vi "PID Initializer.vi"(4 "CANCoder Can IDs":T1, 6 "Cancoder????":bool, 8 "error in":errorcluster, 10 "PIDF":cluster{"P":dbl, "I":dbl, "D":dbl, "F":dbl} {"F" format="%#_13g"; "D" format="%#_13g"; "I" format="%#_13g"; "P" format="%#_13g"}, 11 "Can IDs":T1) -> (0 "error out":errorcluster, 3 "Motors":T7)   [LabVIEW 2020]
uses:
  <vilib>/Rock Robotics/WPI/MotorControl/WPI_MotorControlDeviceRef.ctl
  <vilib>/Rock Robotics/WPI/MotorControl/WPI_MotorControlType.ctl
  <vilib>/Rock Robotics/SystemInterfaces/DIO/FPGA_DIOPWMChannel.ctl
  <vilib>/Rock Robotics/WPI/PWM/WPI_PWMDeadband.ctl
  <vilib>/Rock Robotics/SystemInterfaces/DIO/FPGA_DIOChannel.ctl
  <vilib>/Rock Robotics/WPI/ThirdParty/Phoenix-LabVIEW/Motor Controller/Controls/CTRE_Phoenix_MotorControl_NeutralMode.ctl
  <vilib>/Rock Robotics/WPI/ThirdParty/Phoenix-LabVIEW/Motor Controller/Controls/CTRE_Phoenix_MotorControl_FeedbackDevice_TalonFX.ctl
  <vilib>/Rock Robotics/WPI/ThirdParty/Phoenix-LabVIEW/Motor Controller/Controls/CTRE_Phoenix_MotorControl_RemoteSourceType.ctl
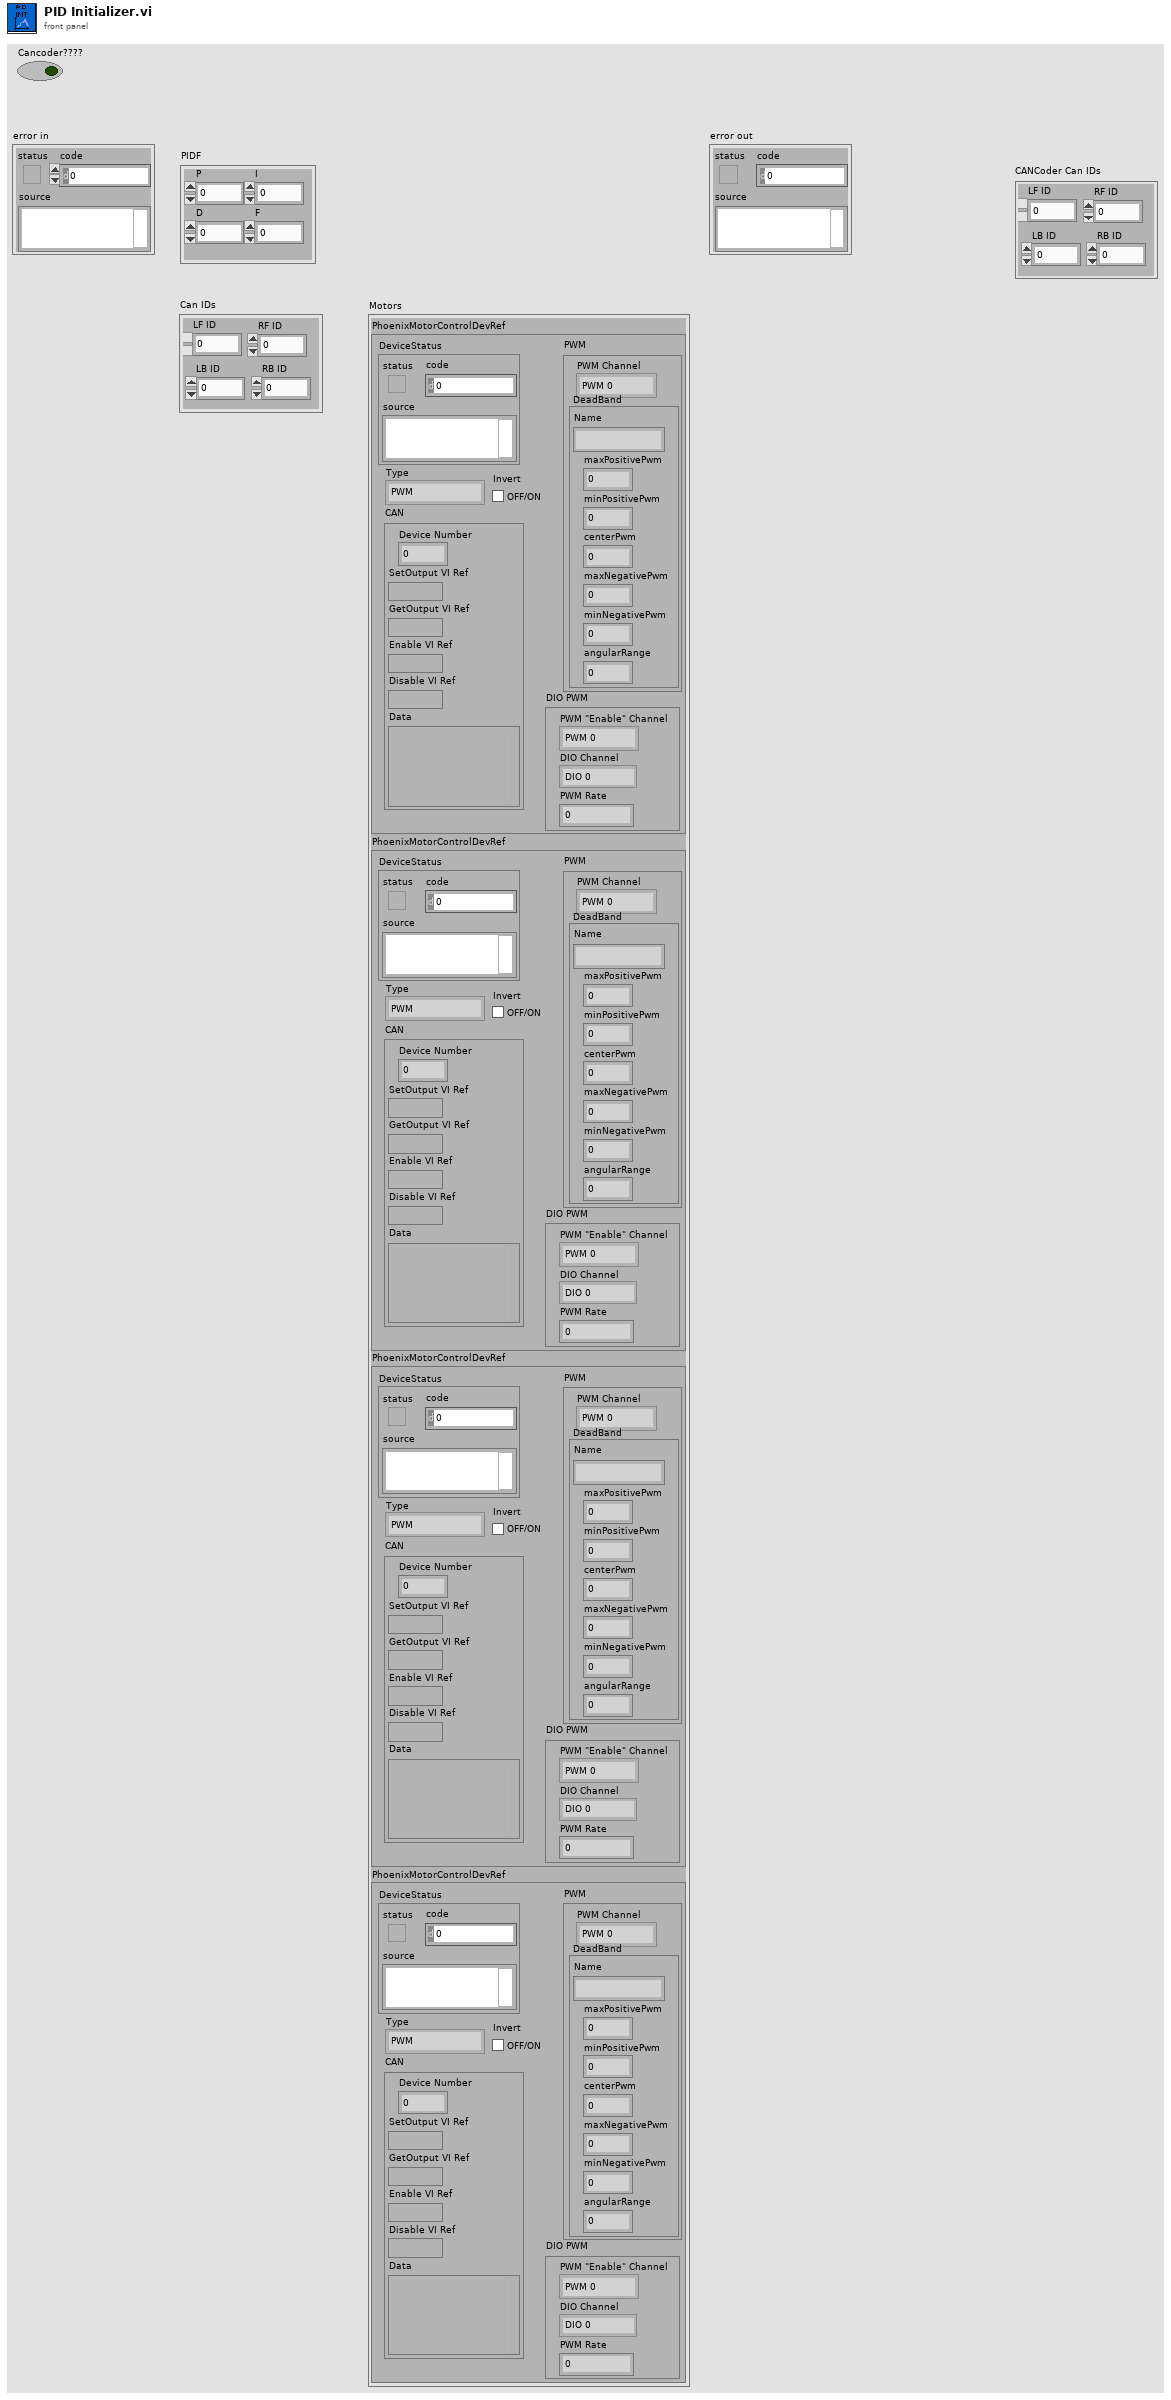
[diagram p1: front panel]
types:
  T1 = cluster{"LF ID":u8, "LB ID":u8, "RF ID":u8, "RB ID":u8}
  T2 = typedef "WPI_MotorControlDeviceRef.ctl" = cluster{"DeviceStatus":errorcluster, "Type":T3, "PWM":cluster{"PWM Channel":T4, "DeadBand":T5}, "CAN":cluster{"Device Number":u8, "SetOutput VI Ref":variant, "GetOutput VI Ref":variant, "Enable VI Ref":variant, "Disable VI Ref":variant, "Data":variant}, "Invert":bool, "DIO PWM":cluster{"PWM \"Enable\" Channel":T4, "DIOChannel":T6, "PWM Rate":dbl}}
  T3 = typedef "WPI_MotorControlType.ctl" = enum16{"PWM", "CAN", "DIO PWM"}
  T4 = typedef "FPGA_DIOPWMChannel.ctl" = enum8{"PWM 0", "PWM 1", "PWM 2", "PWM 3", "PWM 4", "PWM 5", "PWM 6", "PWM 7", "PWM 8", "PWM 9", "PWM MXP 0", "PWM MXP 1", "PWM MXP 2", "PWM MXP 3", "PWM MXP 4", "PWM MXP 5", "PWM MXP 6", "PWM MXP 7", "PWM MXP 8", "PWM MXP 9", "Invalid"}
  T5 = typedef "WPI_PWMDeadband.ctl" = cluster{"Name":string, "maxPositivePwm":i32, "minPositivePwm":i32, "centerPwm":i32, "maxNegativePwm":i32, "minNegativePwm":i32, "angularRange":u16}
  T6 = typedef "FPGA_DIOChannel.ctl" = enum8{"DIO 0", "DIO 1", "DIO 2", "DIO 3", "DIO 4", "DIO 5", "DIO 6", "DIO 7", "DIO 8", "DIO 9", "DIO MXP 0", "DIO MXP 1", "DIO MXP 2", "DIO MXP 3", "DIO MXP 4", "DIO MXP 5", "DIO MXP 6", "DIO MXP 7", "DIO MXP 8", "DIO MXP 9", "DIO MXP 10", "DIO MXP 11", "DIO MXP 12", "DIO MXP 13", "DIO MXP 14", "DIO MXP 15", "SPI Port CS1", "SPI Port CS2", "SPI Port CS3", "SPI Port MISO", "SPI Port MOSI", "Invalid"}
  T7 = cluster{"PhoenixMotorControlDevRef":T2, "PhoenixMotorControlDevRef":T2, "PhoenixMotorControlDevRef":T2, "PhoenixMotorControlDevRef":T2}
  T8 = typedef "CTRE_Phoenix_MotorControl_NeutralMode.ctl" = enum8{"EEPROMSetting", "Override to Coast", "Override to Brake"}
  T9 = typedef "CTRE_Phoenix_MotorControl_RemoteSourceType.ctl" = enum16{"Off", "Talon SRX Selected Sensor", "Pigeon IMU Yaw", "Pigeon IMU Pitch", "Pigeon IMU Roll", "CANifier Quadrature", "CANifier PWM Input 0", "CANifier PWM Input 1", "CANifier PWM Input 2", "CANifier PWM Input 3", "Gadgeteer Pigeon Yaw", "Gadgeteer Pigeon Pitch", "Gadgeteer Pigeon Roll", "CANCoder"}
  T10 = typedef "CTRE_Phoenix_MotorControl_FeedbackDevice_TalonFX.ctl" = i8
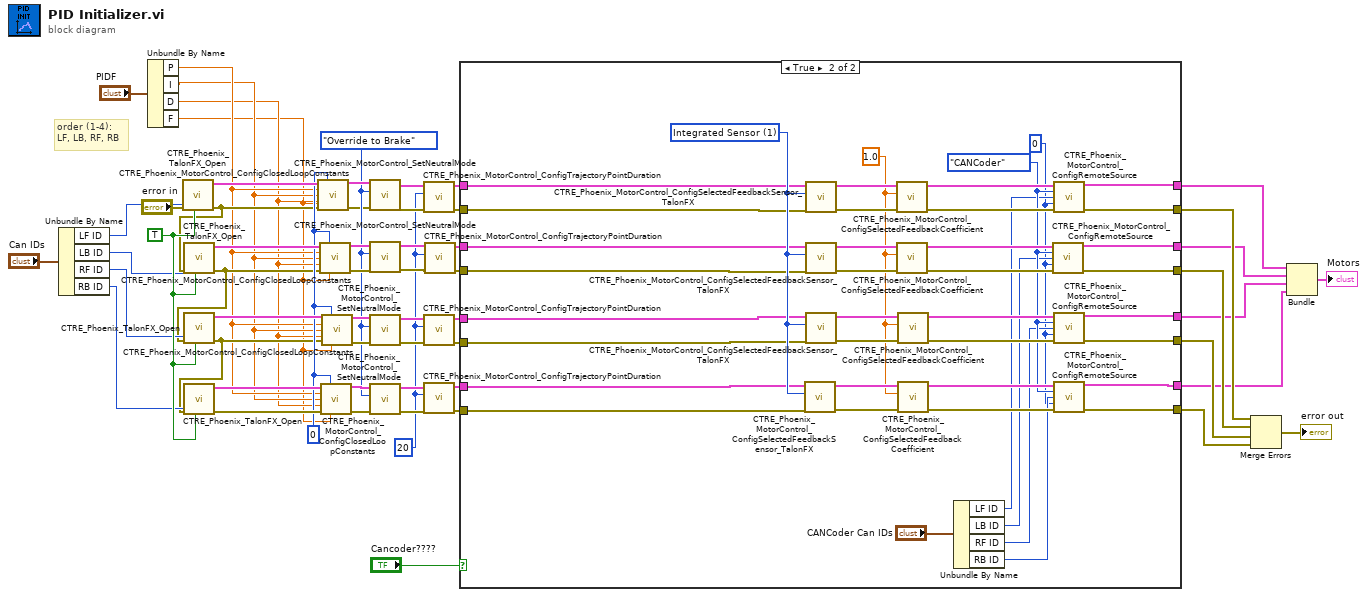
[diagram p0: block diagram]
diagram:
  w19 = 20 ("durationMs")
  w32 = CTRE_Phoenix_MotorControl_NeutralMode."Override to Brake" ("Motor Control Neutral Mode")
  w52 = 0 ("slotIdx")
  w53 = TRUE ("Invert")
  # "order (1-4):\nLF, LB, RF, RB"
  n1 = Unbundle By Name("Can IDs") -> ("LF ID"=w51:u8, "LB ID"=w50:u8, "RF ID"=w49:u8, "RB ID"=w48:u8)
  n2 = Unbundle By Name("PIDF") -> ("P"=w43:dbl, "I"=w42:dbl, "D"=w41:dbl, "F"=w40:dbl)
  n3 = call <vilib>:"CTRE_Phoenix_TalonFX_Open.vi"("Invert"=w53, "error in"="error in", "Device Number"=w51) -> ("error out"=w47:errorcluster, "PhoenixMotorControlDevRef"=w58:T2)  [unwired: 7 in]
  n4 = call <vilib>:"CTRE_Phoenix_TalonFX_Open.vi"("Invert"=w53, "error in"=w47, "Device Number"=w50) -> ("error out"=w46:errorcluster, "PhoenixMotorControlDevRef"=w57:T2)  [unwired: 7 in]
  n5 = call <vilib>:"CTRE_Phoenix_TalonFX_Open.vi"("Invert"=w53, "error in"=w46, "Device Number"=w49) -> ("error out"=w45:errorcluster, "PhoenixMotorControlDevRef"=w56:T2)  [unwired: 7 in]
  n6 = call <vilib>:"CTRE_Phoenix_TalonFX_Open.vi"("Invert"=w53, "error in"=w45, "Device Number"=w48) -> ("error out"=w54:errorcluster, "PhoenixMotorControlDevRef"=w55:T2)  [unwired: 7 in]
  n7 = call <vilib>:"CTRE_Phoenix_MotorControl_ConfigClosedLoopConstants.vi"("PhoenixMotorControlDevRef"=w58, "slotIdx"=w52, "P"=w43, "I"=w42, "D"=w41, "error in (no error)"=w47, "F"=w40) -> ("PhoenixMotorControlDevRef"=w33:T2, "error out"=w31:errorcluster)  [unwired: 7 in]
  n8 = call <vilib>:"CTRE_Phoenix_MotorControl_ConfigClosedLoopConstants.vi"("PhoenixMotorControlDevRef"=w57, "slotIdx"=w52, "P"=w43, "I"=w42, "D"=w41, "error in (no error)"=w46, "F"=w40) -> ("PhoenixMotorControlDevRef"=w37:T2, "error out"=w38:errorcluster)  [unwired: 7 in]
  n9 = call <vilib>:"CTRE_Phoenix_MotorControl_ConfigClosedLoopConstants.vi"("PhoenixMotorControlDevRef"=w55, "slotIdx"=w52, "P"=w43, "I"=w42, "D"=w41, "error in (no error)"=w54, "F"=w40) -> ("PhoenixMotorControlDevRef"=w34:T2, "error out"=w30:errorcluster)  [unwired: 7 in]
  n10 = call <vilib>:"CTRE_Phoenix_MotorControl_ConfigClosedLoopConstants.vi"("PhoenixMotorControlDevRef"=w56, "slotIdx"=w52, "P"=w43, "I"=w42, "D"=w41, "error in (no error)"=w45, "F"=w40) -> ("PhoenixMotorControlDevRef"=w35:T2, "error out"=w36:errorcluster)  [unwired: 7 in]
  n11 = call <vilib>:"CTRE_Phoenix_MotorControl_SetNeutralMode.vi"("error in (no error)"=w31, "Motor Control Neutral Mode"=w32, "PhoenixMotorControlDevRef"=w33) -> ("error out"=w21:errorcluster, "PhoenixMotorControlDevRef"=w20:T2)  [unwired: 7 in]
  n12 = call <vilib>:"CTRE_Phoenix_MotorControl_SetNeutralMode.vi"("error in (no error)"=w38, "Motor Control Neutral Mode"=w32, "PhoenixMotorControlDevRef"=w37) -> ("error out"=w22:errorcluster, "PhoenixMotorControlDevRef"=w23:T2)  [unwired: 7 in]
  n13 = call <vilib>:"CTRE_Phoenix_MotorControl_SetNeutralMode.vi"("error in (no error)"=w36, "Motor Control Neutral Mode"=w32, "PhoenixMotorControlDevRef"=w35) -> ("error out"=w24:errorcluster, "PhoenixMotorControlDevRef"=w25:T2)  [unwired: 7 in]
  n14 = call <vilib>:"CTRE_Phoenix_MotorControl_SetNeutralMode.vi"("error in (no error)"=w30, "Motor Control Neutral Mode"=w32, "PhoenixMotorControlDevRef"=w34) -> ("error out"=w26:errorcluster, "PhoenixMotorControlDevRef"=w27:T2)  [unwired: 7 in]
  n15 = call <vilib>:"CTRE_Phoenix_MotorControl_ConfigTrajectoryPointDuration.vi"("error in"=w21, "durationMs"=w19, "PhoenixMotorControlDevRef"=w20) -> ("error out"=w16:errorcluster, "PhoenixMotorControlDevRef"=w17:T2)  [unwired: 7 in]
  n16 = call <vilib>:"CTRE_Phoenix_MotorControl_ConfigTrajectoryPointDuration.vi"("error in"=w24, "durationMs"=w19, "PhoenixMotorControlDevRef"=w25) -> ("error out"=w12:errorcluster, "PhoenixMotorControlDevRef"=w13:T2)  [unwired: 7 in]
  n17 = call <vilib>:"CTRE_Phoenix_MotorControl_ConfigTrajectoryPointDuration.vi"("error in"=w26, "durationMs"=w19, "PhoenixMotorControlDevRef"=w27) -> ("error out"=w10:errorcluster, "PhoenixMotorControlDevRef"=w11:T2)  [unwired: 7 in]
  n18 = call <vilib>:"CTRE_Phoenix_MotorControl_ConfigTrajectoryPointDuration.vi"("error in"=w22, "durationMs"=w19, "PhoenixMotorControlDevRef"=w23) -> ("error out"=w14:errorcluster, "PhoenixMotorControlDevRef"=w15:T2)  [unwired: 7 in]
  n19 = case shown="True" "Cancoder????" {
    tunnel: w17 -> [w66 w97]
    tunnel: w16 -> [w65 w96]
    tunnel: w15 -> [w64 w95]
    tunnel: w14 -> [w63 w94]
    tunnel: w13 -> [w62 w93]
    tunnel: w12 -> [w61 w92]
    tunnel: w11 -> [w60 w91]
    tunnel: w10 -> [w59 w90]
    tunnel: [w66 w87] -> w9
    tunnel: [w65 w86] -> w8
    tunnel: [w64 w83] -> w7
    tunnel: [w63 w82] -> w6
    tunnel: [w62 w79] -> w5
    tunnel: [w61 w78] -> w4
    tunnel: [w60 w75] -> w3
    tunnel: [w59 w74] -> w2
    frame False {
    }
    frame True {
      w68 = u32 0 ("Source Index (0/1)")
      w73 = CTRE_Phoenix_MotorControl_RemoteSourceType."CANCoder" ("Remote Device Type")
      w98 = 1.0 ("coefficient")
      w107 = T10 1 items=["Integrated Sensor"=1, "Sensor Sum (S0 + S1)"=9, "Sensor Difference (D0 - D1)"=10, "Remote Source 0"=11, "Remote Source 1"=12, "None"=14, "Software Emulated"=15] ("Talon FX Feedback Device")
      n20 = call <vilib>:"CTRE_Phoenix_MotorControl_ConfigSelectedFeedbackSensor_TalonFX.vi"("error in (no error)"=w90, "Talon FX Feedback Device"=w107, "PhoenixMotorControlDevRef"=w91) -> ("error out"=w99:errorcluster, "PhoenixMotorControlDevRef"=w100:T2)  [unwired: 7 in]
      n21 = call <vilib>:"CTRE_Phoenix_MotorControl_ConfigSelectedFeedbackSensor_TalonFX.vi"("error in (no error)"=w96, "Talon FX Feedback Device"=w107, "PhoenixMotorControlDevRef"=w97) -> ("error out"=w105:errorcluster, "PhoenixMotorControlDevRef"=w106:T2)  [unwired: 7 in]
      n22 = call <vilib>:"CTRE_Phoenix_MotorControl_ConfigSelectedFeedbackSensor_TalonFX.vi"("error in (no error)"=w94, "Talon FX Feedback Device"=w107, "PhoenixMotorControlDevRef"=w95) -> ("error out"=w103:errorcluster, "PhoenixMotorControlDevRef"=w104:T2)  [unwired: 7 in]
      n23 = call <vilib>:"CTRE_Phoenix_MotorControl_ConfigSelectedFeedbackSensor_TalonFX.vi"("error in (no error)"=w92, "Talon FX Feedback Device"=w107, "PhoenixMotorControlDevRef"=w93) -> ("error out"=w101:errorcluster, "PhoenixMotorControlDevRef"=w102:T2)  [unwired: 7 in]
      n24 = call <vilib>:"CTRE_Phoenix_MotorControl_ConfigSelectedFeedbackCoefficient.vi"("error in (no error)"=w105, "coefficient"=w98, "PhoenixMotorControlDevRef"=w106) -> ("error out"=w88:errorcluster, "PhoenixMotorControlDevRef"=w89:T2)  [unwired: 7 in]
      n25 = call <vilib>:"CTRE_Phoenix_MotorControl_ConfigSelectedFeedbackCoefficient.vi"("error in (no error)"=w103, "coefficient"=w98, "PhoenixMotorControlDevRef"=w104) -> ("error out"=w84:errorcluster, "PhoenixMotorControlDevRef"=w85:T2)  [unwired: 7 in]
      n26 = call <vilib>:"CTRE_Phoenix_MotorControl_ConfigSelectedFeedbackCoefficient.vi"("error in (no error)"=w101, "coefficient"=w98, "PhoenixMotorControlDevRef"=w102) -> ("error out"=w80:errorcluster, "PhoenixMotorControlDevRef"=w81:T2)  [unwired: 7 in]
      n27 = call <vilib>:"CTRE_Phoenix_MotorControl_ConfigSelectedFeedbackCoefficient.vi"("error in (no error)"=w99, "coefficient"=w98, "PhoenixMotorControlDevRef"=w100) -> ("error out"=w76:errorcluster, "PhoenixMotorControlDevRef"=w77:T2)  [unwired: 7 in]
      n28 = Unbundle By Name("CANCoder Can IDs") -> ("LF ID"=w72:u8, "LB ID"=w71:u8, "RF ID"=w70:u8, "RB ID"=w69:u8)
      n29 = call <vilib>:"CTRE_Phoenix_MotorControl_ConfigRemoteSource.vi"("PhoenixMotorControlDevRef"=w85, "Remote Device Type"=w73, "Remote Device ID"=w71, "Source Index (0/1)"=w68, "error in (no error)"=w84) -> ("PhoenixMotorControlDevRef"=w83:T2, "error out"=w82:errorcluster)  [unwired: 9 in]
      n30 = call <vilib>:"CTRE_Phoenix_MotorControl_ConfigRemoteSource.vi"("PhoenixMotorControlDevRef"=w89, "Remote Device Type"=w73, "Remote Device ID"=w72, "Source Index (0/1)"=w68, "error in (no error)"=w88) -> ("PhoenixMotorControlDevRef"=w87:T2, "error out"=w86:errorcluster)  [unwired: 9 in]
      n31 = call <vilib>:"CTRE_Phoenix_MotorControl_ConfigRemoteSource.vi"("PhoenixMotorControlDevRef"=w81, "Remote Device Type"=w73, "Remote Device ID"=w70, "Source Index (0/1)"=w68, "error in (no error)"=w80) -> ("PhoenixMotorControlDevRef"=w79:T2, "error out"=w78:errorcluster)  [unwired: 9 in]
      n32 = call <vilib>:"CTRE_Phoenix_MotorControl_ConfigRemoteSource.vi"("PhoenixMotorControlDevRef"=w77, "Remote Device Type"=w73, "Remote Device ID"=w69, "Source Index (0/1)"=w68, "error in (no error)"=w76) -> ("PhoenixMotorControlDevRef"=w75:T2, "error out"=w74:errorcluster)  [unwired: 9 in]
    }
  }
  n33 = Merge Errors(w8, w6, w4, w2) -> (→"error out":errorcluster)
  n34 = Bundle("PhoenixMotorControlDevRef"=w9, "PhoenixMotorControlDevRef"=w7, "PhoenixMotorControlDevRef"=w5, "PhoenixMotorControlDevRef"=w3) -> (→"Motors":T7)  [unwired: 1 in]
